vi "FormXErrorCluster.vi"(8 "Help Topic":T2, 9 "Help File":T2, 10 "Details":T2, 11 "Error":T2) -> (3 "XError Cluster":T1)   [LabVIEW 2020, in "NI_XNodeSupport.lvlib"]
uses:
  NI_XNodeSupport.lvlib
  XNodeString.ctl
  XNodeError3.ctl
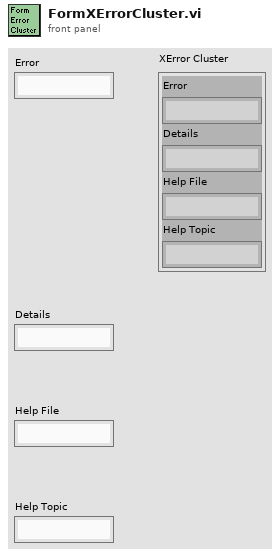
[diagram p1: front panel]
types:
  T1 = typedef "NI_XNodeSupport.lvlib/XNodeError3.ctl" = cluster{"Error":T2, "Details":T2, "Help File":T2, "Help Topic":T2}
  T2 = typedef "NI_XNodeSupport.lvlib/XNodeString.ctl" = string
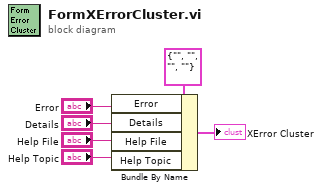
[diagram p0: block diagram]
diagram:
  n1 = Bundle By Name(cluster=T1 {"Error"="", "Details"="", "Help File"="", "Help Topic"=""} ("Error Cluster"), "Error"="Error", "Details"="Details", "Help File"="Help File", "Help Topic"="Help Topic") -> (→"XError Cluster":T1)
